vi "MP-285 Init.vi"(2 "Input: Error Cluster":errorcluster, 3 "Timeout (msec)":u32=200, 4 "Serial port # \n(COM1 - #1)!!!":u16=5) -> (0 "error out":errorcluster={"status"=TRUE, "code"=-1073807343, "source"="Old VISA Open in MP-285 Init.vi"}, 1 "reference out":refnum<visa-resource-name>="ASRL0::INSTR")   [LabVIEW 2010]
doc: "This VI sets up the serial port and VISA for use with the MVP2001 controller\nThe MVP2001 node number is stored in the user data input of the property node.\nnote: The MVP2001 requires that, the flow control is set to \"none\""
panel:
  out "VISA resource":string="ASRL0::INSTR"
  in  "VISA session IN":refnum<visa-resource-name>
  in  "Serial Settings:\nSerial End Mode for Writes":u16(ring) items=["None", "LastBit", "TermChar", "Break"]
  in  "Serial Settings:\nSerial End Mode for Reads":u16(ring) items=["None", "LastBit", "TermChar"]
  in  "Flow control":enum16{"None", "XON/XOFF", "RTS/CTS"}(ring)
  in  "Parity":enum16{"None", "Odd", "Even", "Mark", "Space"}(ring)
  in  "Stop bits":bool
  in  "data bits (8)":u16=8
  in  "baud rate (9600)":u32=9600
  # "_____________________________________"
  # "Use this settings to define \nparameters \"by definition\"\n(If the inputs is NOT wired)"
  # "Windows:\nCom1 - #1;\nCom2 - #2;\nCom3 - #3;\nCom4 - #4."
  # "_______________________________________"
  # "This settings should be changed\nONLY if the SUTTER change the\n     default hardware settings."
  # "___________________\n\nTest Indicators/Controls:"
  # "___________________"
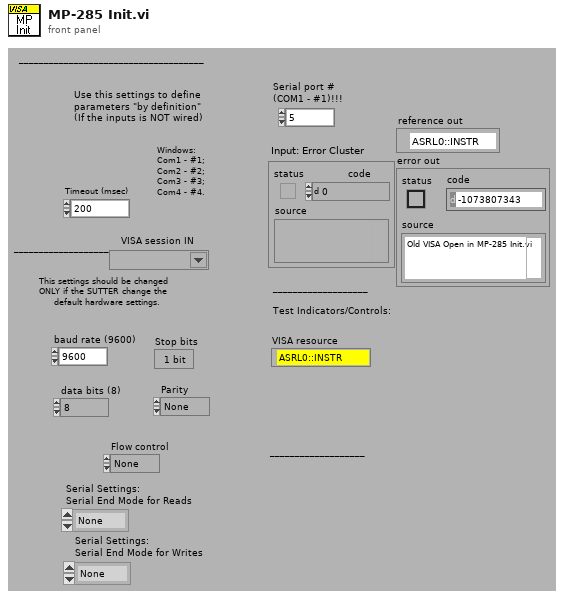
[diagram p1: front panel]
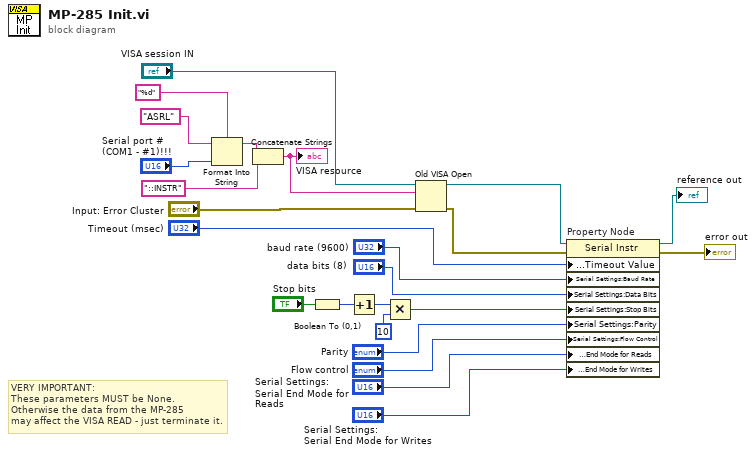
[diagram p0: block diagram]
diagram:
  # "VERY IMPORTANT:\nThese parameters MUST be None.\nOtherwise the data from the MP-285\nmay affect the VISA READ - just terminate it."
  n1 = Format Into String(format string="%d", initial string="ASRL", "Serial port # \n(COM1 - #1)!!!") -> (resulting string=w7:string)  [unwired: 1 in, 1 out]
  n2 = Concatenate Strings(w7, "::INSTR") -> (w10:string)
  "VISA resource" <- w10
  n3 = Boolean To (0,1)(Boolean="Stop bits") -> (0, 1=w22:i16)
  n4 = Increment(x=w22) -> (x+1=w21:i16)
  n5 = Multiply(x=w21, y=u16 10) -> (x*y=w15:u16)
  n6 = Old VISA Open(8:"Input: Error Cluster", 10:w10, 11:"VISA session IN") -> (0:w2:errorcluster, 3:w1:refnum<visa-resource-name>)  [unwired: 2 out]
  n7 = property on="Property Node" class="Serial Instr"(reference=w1, error in=w2, "General Settings:Timeout Value"="Timeout (msec)", "Serial Settings:Baud Rate"="baud rate (9600)", "Serial Settings:Data Bits"="data bits (8)", "Serial Settings:Stop Bits"=w15, "Serial Settings:Parity"="Parity", "Serial Settings:Flow Control"="Flow control", "Serial Settings:End Mode for Reads"="Serial Settings:\nSerial End Mode for Reads", "Serial Settings:End Mode for Writes"="Serial Settings:\nSerial End Mode for Writes") -> (reference out=→"reference out":refnum<visa-resource-name>, error out=→"error out":errorcluster)
